vi "X_2.46_IO_Ohms.vi"() -> ()   [LabVIEW 2022 SP3]
uses:
  <vilib>/Utility/file.llb/Read Delimited Spreadsheet (DBL).vi
  <vilib>/Utility/file.llb/Write Delimited Spreadsheet (string).vi
panel:
  in  "Save":bool
  out "Saved Path":string
  in  "stop":bool
  in  "Clear Graf":bool
  out "R Data":dbl[](array[numeric])
  in  "OK Button":bool
  out "XY Graph":cluster{"array":dbl[], "all rows":dbl[]}(graph)
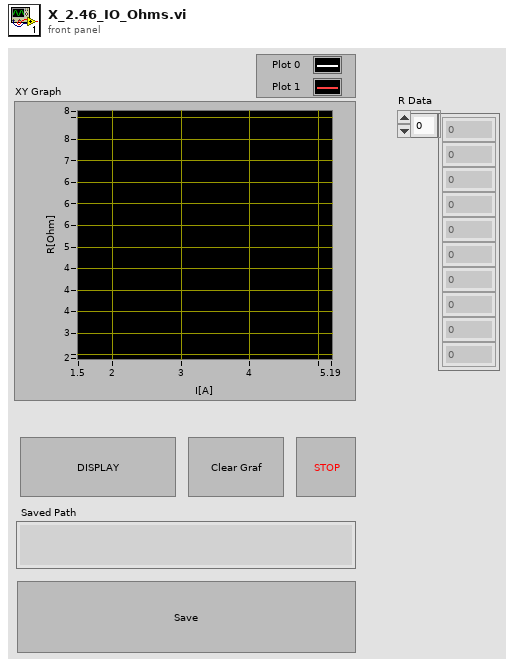
[diagram p1: front panel]
types:
  T1 = cluster{"all rows":dbl[], "initialized array":dbl[]}
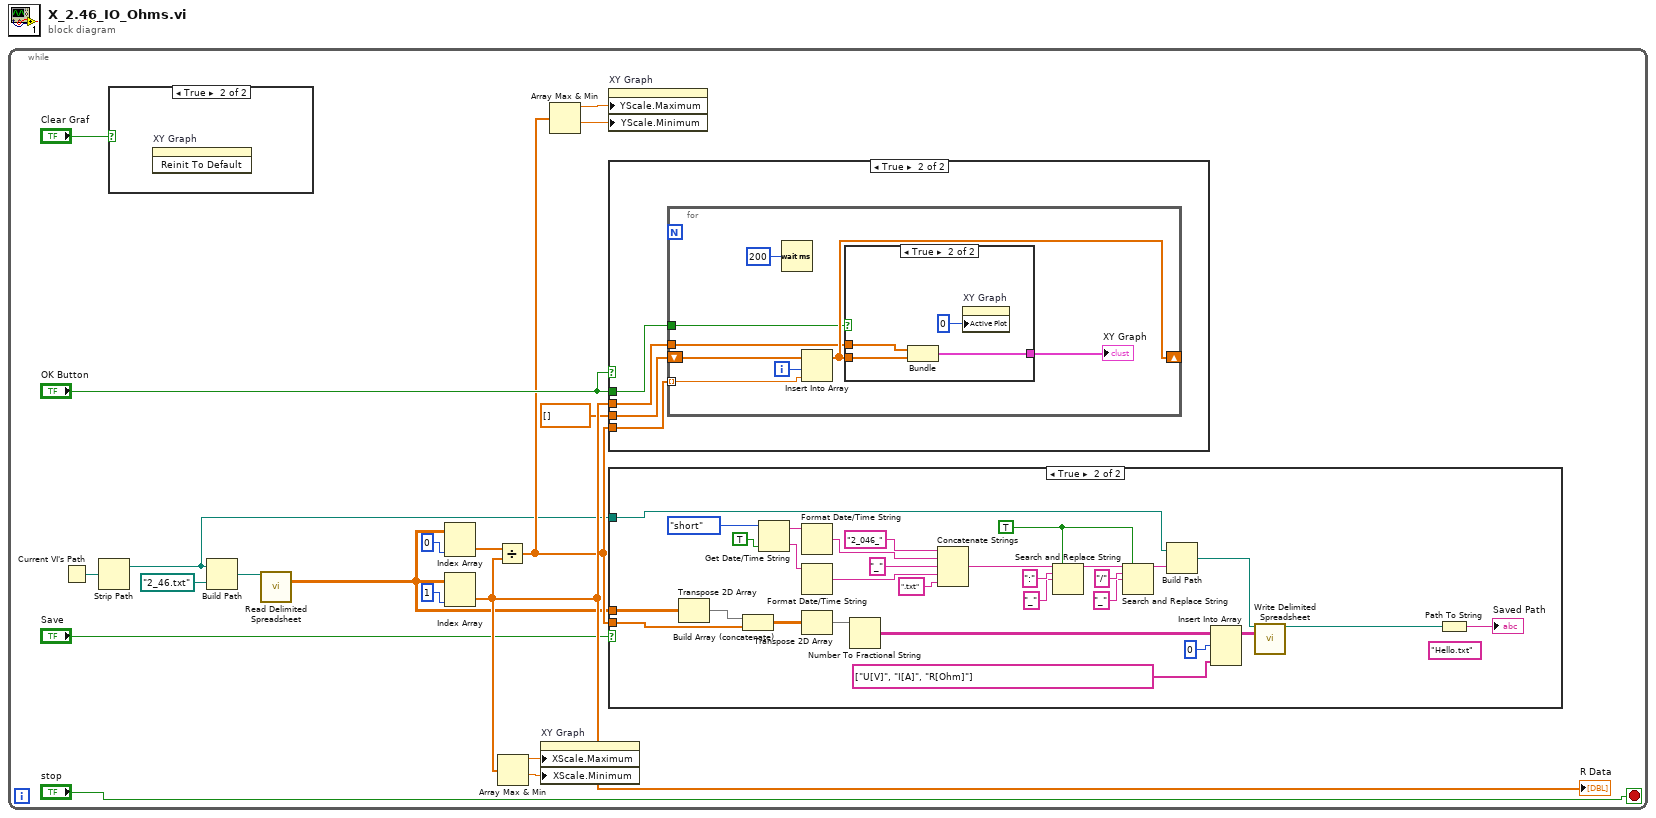
[diagram p0: block diagram]
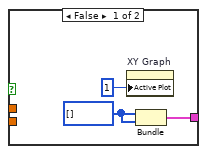
[diagram p5: hidden frame]
diagram:
  n1 = while {
    stop <- "stop" stop-if-true
    n2 = Current VI's Path() -> (path=w14:path)
    n3 = Strip Path(path=w14) -> (stripped path=w2:path)  [unwired: 1 out]
    n4 = case shown="True" "Clear Graf" {
      frame False {
      }
      frame True {
        n5 = invoke on="XY Graph" class="XYGraph (strict)" method="Reinit To Default"() -> ()  [unwired: 3 in, 3 out]
      }
    }
    n6 = Build Path(base path=w2, name or relative path=path "2_46.txt") -> (appended path=w15:path)
    n7 = call-poly <vilib>:"Read Delimited Spreadsheet.vi"("file path (dialog if empty)"=w15) -> ("all rows"=w3:dbl[][])  [unwired: 9 in, 5 out]
    n8 = Index Array(array=w3, index (col)=0 ("disabled index (col)")) -> (element=w19:dbl[])  [unwired: 1 in]
    n9 = Index Array(array=w3, index (col)=1 ("disabled index (col)")) -> (element=w18:dbl[])  [unwired: 1 in]
    "R Data" <- w18
    n10 = Divide(x=w19, y=w18) -> (x/y=w4:dbl[])
    n11 = Array Max & Min(array=w18) -> (max value=w16:dbl, min value=w17:dbl)  [unwired: 2 out]
    n12 = property on="XY Graph" class="XYGraph (strict)"("XScale.Maximum"=w16, "XScale.Minimum"=w17) -> ()  [unwired: 2 in, 2 out]
    n13 = Array Max & Min(array=w4) -> (max value=w9:dbl, min value=w8:dbl)  [unwired: 2 out]
    n14 = property on="XY Graph" class="XYGraph (strict)"("YScale.Maximum"=w9, "YScale.Minimum"=w8) -> ()  [unwired: 2 in, 2 out]
    n15 = case shown="True" "OK Button" {
      tunnel: w18 -> [_ w53]
      tunnel: dbl[] [] ("initialized array") -> [_ w52]
      tunnel: w4 -> [_ w51]
      tunnel: "OK Button" -> [_ w50]
      frame False {
      }
      frame True {
        n16 = for {
          shift-right: [w58] -> _
          shift-left: w52 -> [w59]
          tunnel: w53 -> [w57]
          tunnel: w51 -> [w56] mode=indexing
          tunnel: w50 -> [w54]
          i -> [w60]
          n17 = Wait (ms)(milliseconds to wait=u32 200) -> ()  [unwired: 1 out]
          n18 = Insert Into Array(array=w59, index=w60, new element=w56) -> (w58:dbl[])
          n19 = case shown="True" w54 {
            tunnel: w58 -> [_ w68]
            tunnel: w57 -> [_ w67]
            tunnel: [w63 w66] -> w55
            frame False {
              w64 = i32[] []
              n20 = property on="XY Graph" class="XYGraph (strict)"("Active Plot"=u32 1) -> ()  [unwired: 2 in, 2 out]
              n21 = Bundle(w64, w64) -> (w63:cluster{i32[], i32[]})  [unwired: 1 in]
            }
            frame True {
              n22 = Bundle("all rows"=w67, "initialized array"=w68) -> (w66:T1)  [unwired: 1 in]
              n23 = property on="XY Graph" class="XYGraph (strict)"("Active Plot"=u32 0) -> ()  [unwired: 2 in, 2 out]
            }
          }
          "XY Graph" <- w55
        }
      }
    }
    n24 = case shown="True" "Save" {
      tunnel: w4 -> [_ w49]
      tunnel: w3 -> [_ w48]
      tunnel: w2 -> [_ w32]
      frame False {
      }
      frame True {
        w25 = TRUE
        (unwired) "Hello.txt" ("concatenated string")
        n25 = Transpose 2D Array(2D array=w48) -> (transposed array=w47:dbl[][])
        n26 = Build Array (concatenate)(w47, w49) -> (w46:dbl[][])
        n27 = Get Date/Time String(date format (0)=enum16{"short", "long", "abbreviated"}."short", want seconds? (F)=TRUE) -> (date string=w36:string, time string=w40:string)  [unwired: 1 in]
        n28 = Format Date/Time String(time format string (%c)=w36) -> (date/time string=w35:string)  [unwired: 2 in]
        n29 = Format Date/Time String(time format string (%c)=w40) -> (date/time string=w37:string)  [unwired: 2 in]
        n30 = Transpose 2D Array(2D array=w46) -> (transposed array=w45:dbl[][])
        n31 = Number To Fractional String(number=w45) -> (F-format string=w44:string[][])  [unwired: 3 in]
        n32 = Concatenate Strings("2_046_" ("string"), w35, "_", w37, ".txt" ("string")) -> (w28:string)
        n33 = Search and Replace String(replace all?=w25, input string=w28, search string=":", replace string="_" ("replace string (\"\")")) -> (result string=w27:string)  [unwired: 4 in, 3 out]
        n34 = Search and Replace String(replace all?=w25, input string=w27, search string="/", replace string="_" ("replace string (\"\")")) -> (result string=w22:string)  [unwired: 4 in, 3 out]
        n35 = Build Path(base path=w32, name or relative path=w22) -> (appended path=w31:path)
        n36 = Insert Into Array(array=w44, index (row)=0 ("disabled index (col)"), new element=string[] ["U[V]", "I[A]", "R[Ohm]"] ("new element/subarray")) -> (w41:string[][])  [unwired: 1 in]
        n37 = call-poly <vilib>:"Write Delimited Spreadsheet.vi"("file path (dialog if empty)"=w31, "2D data"=w41) -> ("new file path (Not A Path if cancelled)"=w21:path)  [unwired: 12 in, 1 out]
        n38 = Path To String(path=w21) -> (string=→"Saved Path":string)
      }
    }
  }
